vi "SetPieceSquares.vi"(8 "error in (no error)":errorcluster, 11 "object in":refnum<class "Board.lvclass">) -> (0 "error out":errorcluster, 3 "object out":refnum<class "Board.lvclass">)   [LabVIEW 2020, in "Board.lvclass"]
uses:
  Board.lvclass
  Pieces/Piece.lvclass
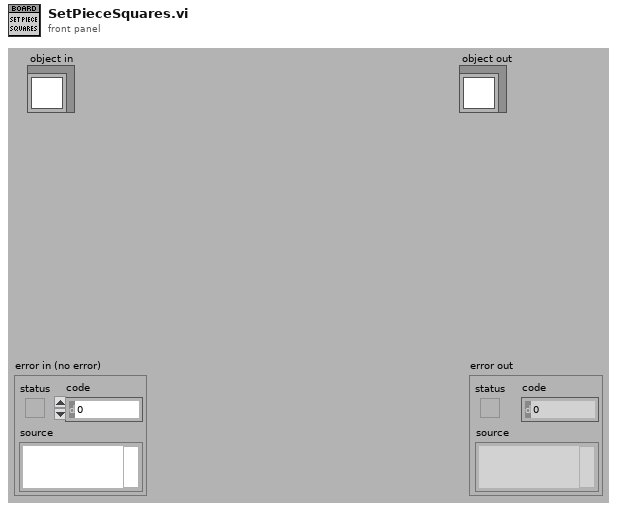
[diagram p1: front panel]
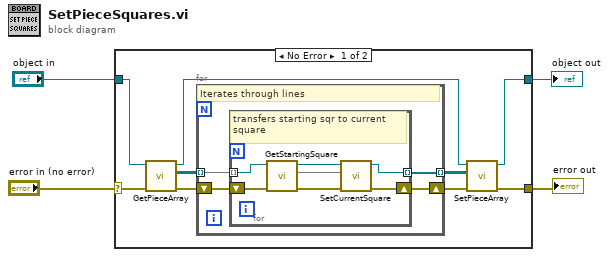
[diagram p0: block diagram]
diagram:
  n1 = case shown="No Error" "error in (no error)" {
    selector: "error in (no error)" -> [w13 w26]
    tunnel: [w8 w26] -> w3
    tunnel: [w6 w25] -> w1
    tunnel: "object in" -> [w12 w25]
    frame No Error {
      n2 = call "GetPieceArray.vi"("error in (no error)"=w13, "object in"=w12) -> ("error out"=w11:errorcluster, "pieceArray"=w10:refnum<class "Piece.lvclass">[][], "object out"=w7:refnum<class "Board.lvclass">)  [unwired: 7 in]
      n3 = for {
        shift-right: [w15] -> w9
        shift-left: w11 -> [w17]
        tunnel: w10 -> [w16] mode=indexing
        tunnel: [w14] -> w5 mode=indexing
        # "Iterates through lines"
        n4 = for {
          shift-right: [w19] -> w15
          shift-left: w17 -> [w24]
          tunnel: w16 -> [w23] mode=indexing
          tunnel: [w18] -> w14 mode=indexing
          # "transfers starting sqr to current square"
          n5 = call "GetStartingSquare.vi"("error in (no error)"=w24, "object in"=w23) -> ("error out"=w20:errorcluster, "startingSquare"=w21:map{string, i32}, "object out"=w22:refnum<class "Piece.lvclass">)  [unwired: 7 in]
          n6 = call "SetCurrentSquare.vi"("error in (no error)"=w20, "currentSquare"=w21, "object in"=w22) -> ("error out"=w19:errorcluster, "object out"=w18:refnum<class "Piece.lvclass">)  [unwired: 7 in]
        }
      }
      n7 = call "SetPieceArray.vi"("error in (no error)"=w9, "pieceArray"=w5, "object in"=w7) -> ("error out"=w8:errorcluster, "object out"=w6:refnum<class "Board.lvclass">)  [unwired: 7 in]
    }
    frame Error {
    }
  }
  "error out" <- w3
  "object out" <- w1
